vi "Frame.Dialog.vi"(6 "Signals":T1[](array[typedef]) {"Byte Order" items=["Little Endian", "Big Endian"]; "Data Type" items=["Signed", "Unsigned", "IEEE Float"]}, 7 "Show Name&ID":bool=TRUE, 8 "error in (no error)":errorcluster, 9 "ID":u16=1 caption="ID/Address" min=1 format="%.0x", 10 "Existing PIDs":string[](array[string]), 11 "Name":string) -> (0 "error out":errorcluster, 1 "ID out":u16=1 min=1 format="%.0x", 2 "Cancel PID?":bool, 3 "Name out":string, 4 "Signals out":T1[](array[typedef]) {"Byte Order" items=["Little Endian", "Big Endian"]; "Data Type" items=["Signed", "Unsigned", "IEEE Float"]})   [LabVIEW 2024, in "Diagnostics Addon System Explorer.lvlib"]
uses:
  Diagnostics Addon System Explorer.lvlib
  Addon Shared/Types/Signal.ctl
  <vilib>/NI/AMC/Create Single Message.vi
  <vilib>/NI/AMC/Update Message Routing Info.vi
  <vilib>/NI/AMC/Read Termination Message.vi
  Addon Shared/SubVIs/Constants.vi
  <vilib>/NI/AMC/Globals.vi
  <vilib>/NI/AMC/Send Message.vi
  Addon Shared/Diagnostics Addon Shared.lvlib
  <vilib>/NI/AMC/AMC.lvlib
panel:
  in  "Add":bool
  in  "Header":cluster{"Section Name":string}={"Section Name"="Frame Settings"}
  in  "SHDocVw.IWebBrowser":refnum<k7>(container)
  in  "Default":dbl format="%g"
  in  "Units":string
  in  "Endian":u8(ring) items=["Little", "Big"]
  in  "Datatype":u8(ring)=1 items=["Signed", "Unsigned", "Float"]
  in  "Remove":bool
  in  "Cancel":bool
  in  "OK":bool
  in  "Maximum":dbl=255.0 format="%g"
  in  "Minimum":dbl format="%g"
  in  "Offset":dbl format="%g"
  in  "Factor":dbl=1.0 format="%g"
  in  "Length":u32=8
  in  "Start Bit":u32
  in  "Signal Name":string
  in  "Signals":i32(listbox)
  in  "Cancel PID":bool
  in  "Apply":bool
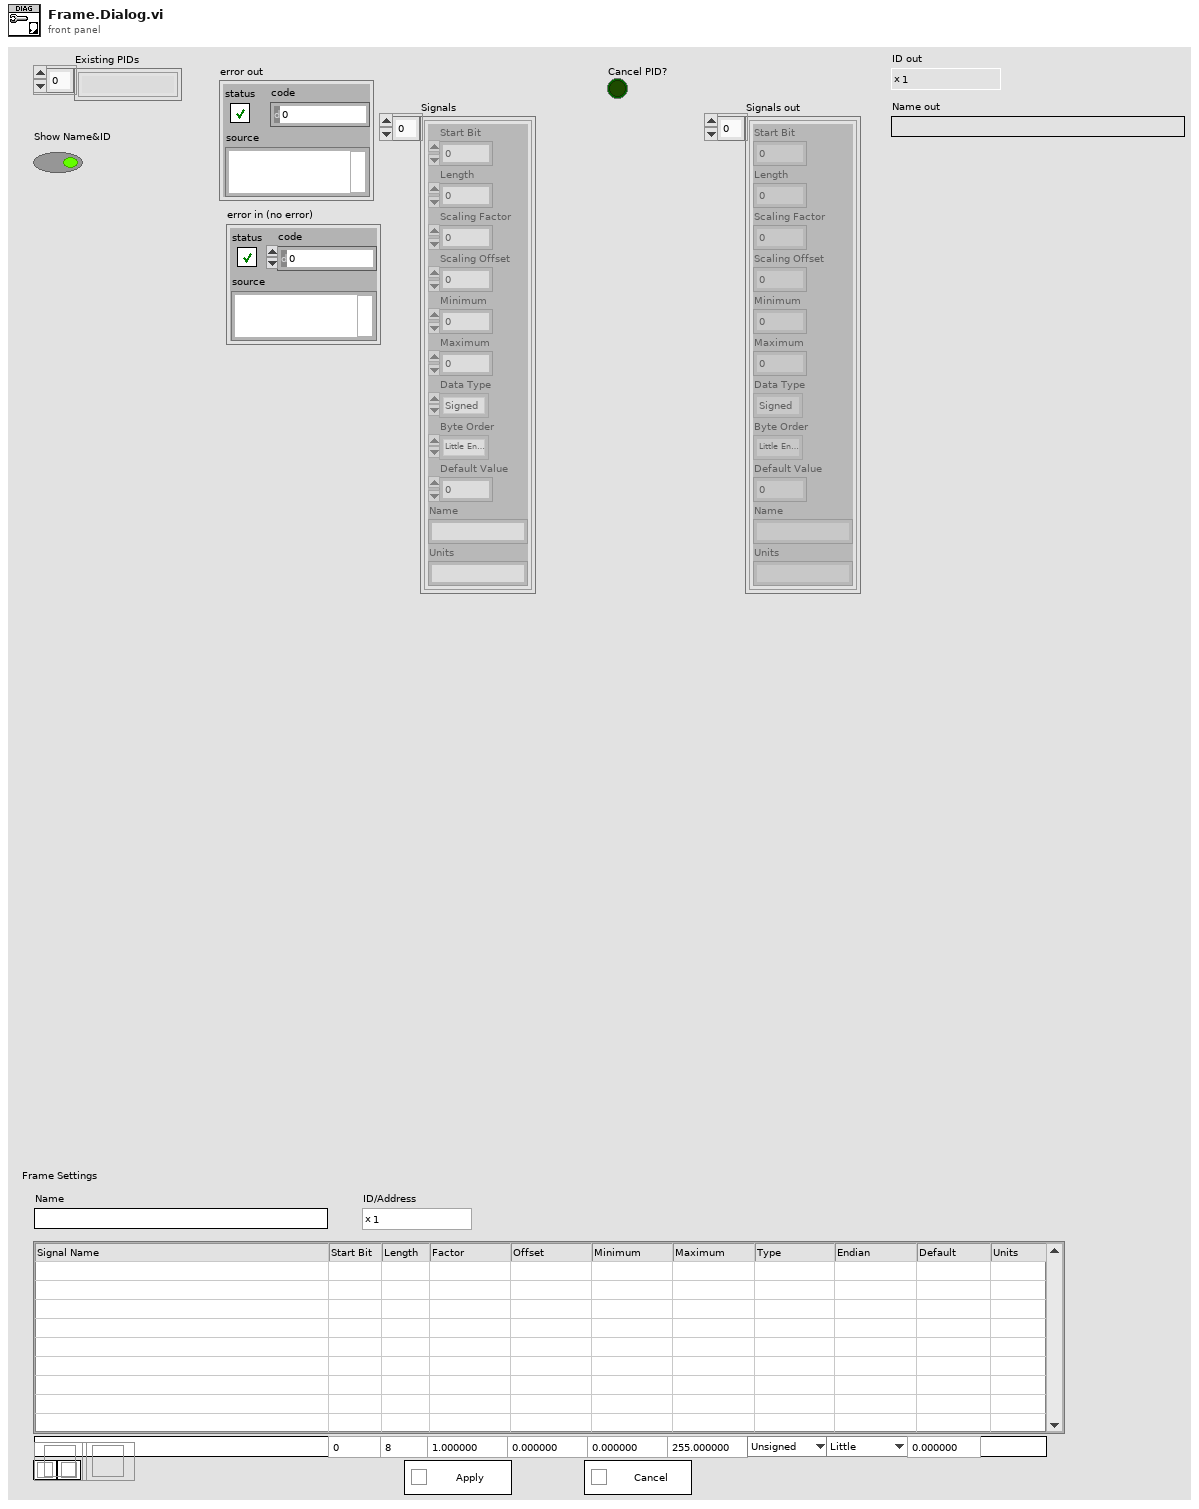
[diagram p1: front panel]
types:
  T1 = typedef "Diagnostics Addon Shared.lvlib/Signal.ctl" = cluster{"Start Bit":u32, "Length":u32, "Scaling Factor":dbl, "Scaling Offset":dbl, "Minimum":dbl, "Maximum":dbl, "Data Type":u32, "Byte Order":u32, "Default Value":dbl, "Name":string, "Units":string}
  T2 = cluster{"NewControlRefs":refnum<vi>[], "Add":refnum<vi>, "Listbox":refnum<vi>, "Remove":refnum<vi>, "Apply":refnum<vi>, "Cancel PID":refnum<vi>}
  T3 = typedef "AMC.lvlib/Message Queue.ctl" = refnum<queue>
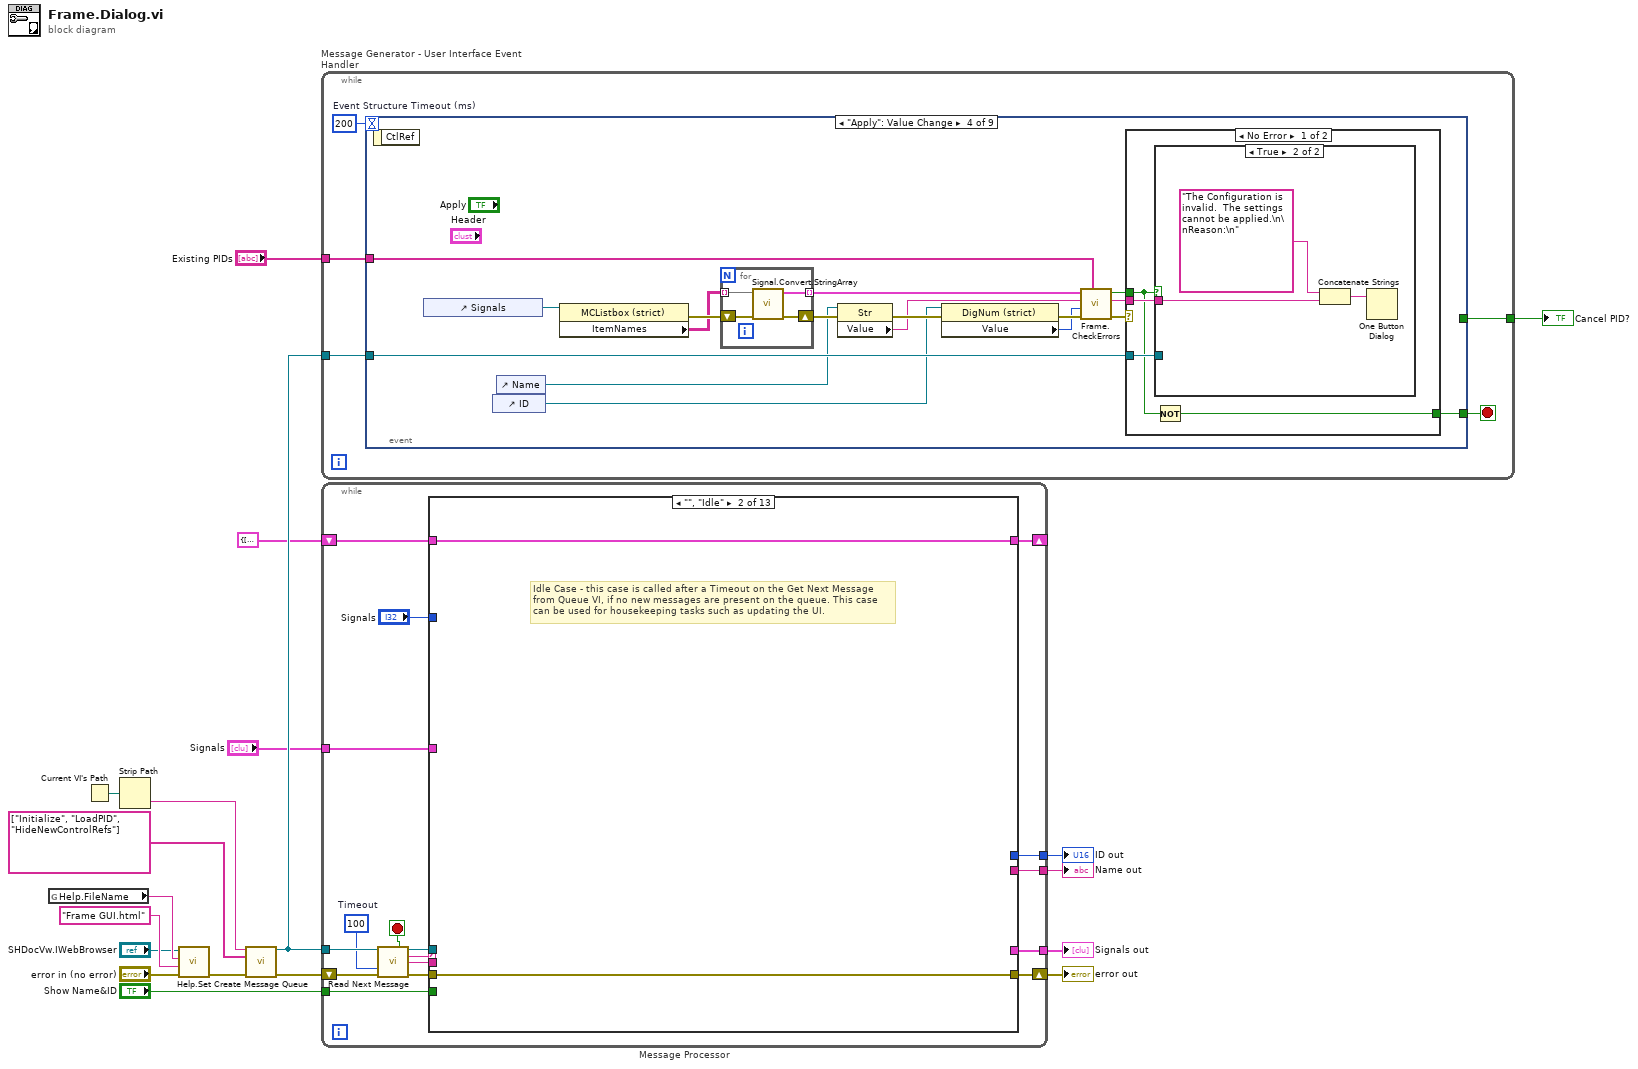
[diagram p0: block diagram]
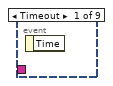
[diagram p2: hidden frame]
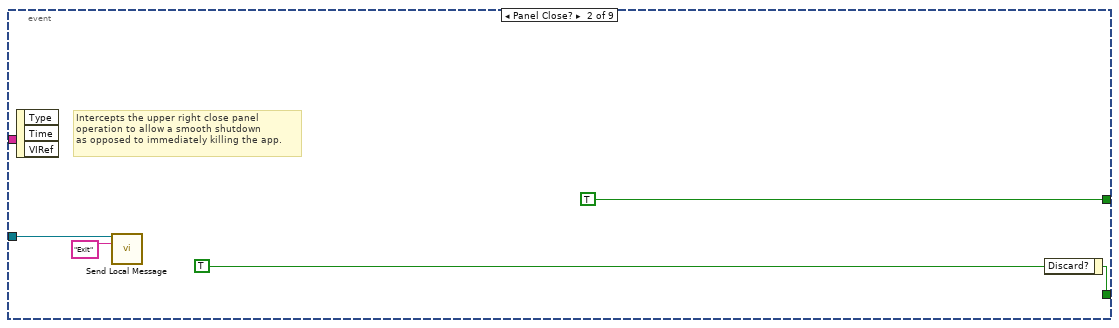
[diagram p3: hidden frame]
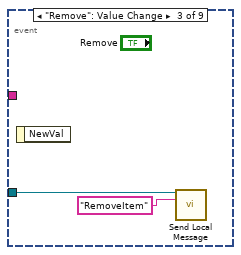
[diagram p4: hidden frame]
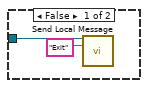
[diagram p5: hidden frame]
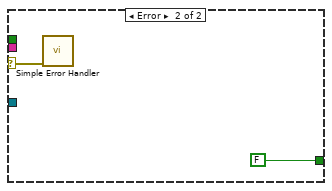
[diagram p6: hidden frame]
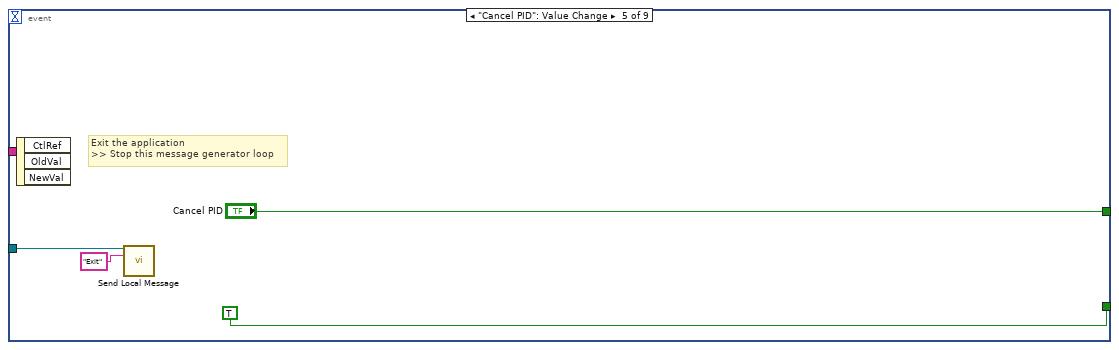
[diagram p7: hidden frame]
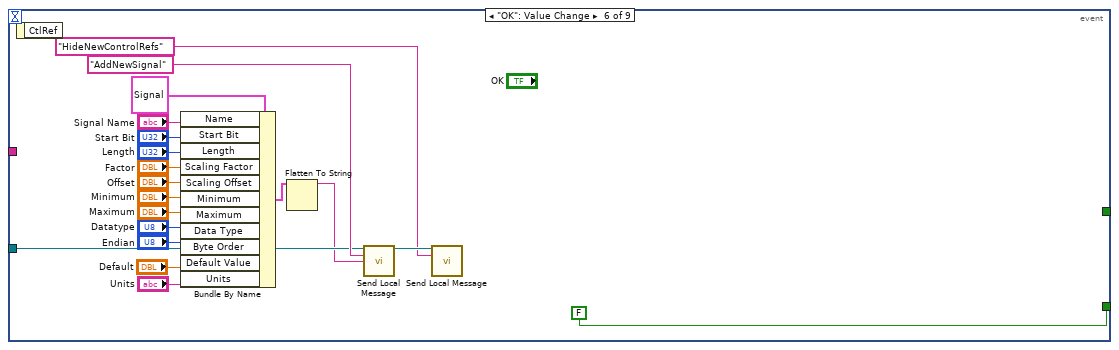
[diagram p8: hidden frame]
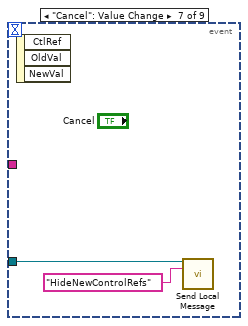
[diagram p9: hidden frame]
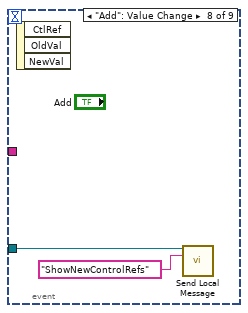
[diagram p10: hidden frame]
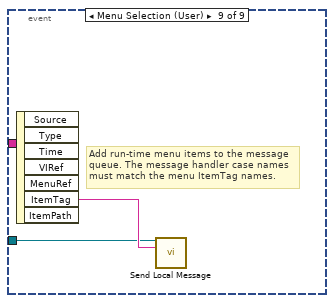
[diagram p11: hidden frame]
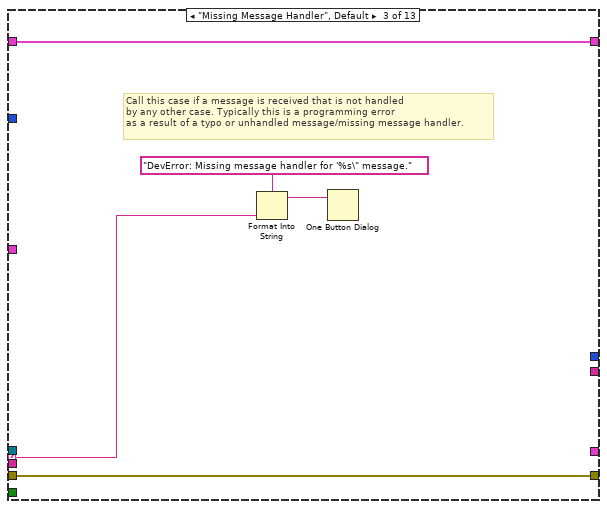
[diagram p13: hidden frame]
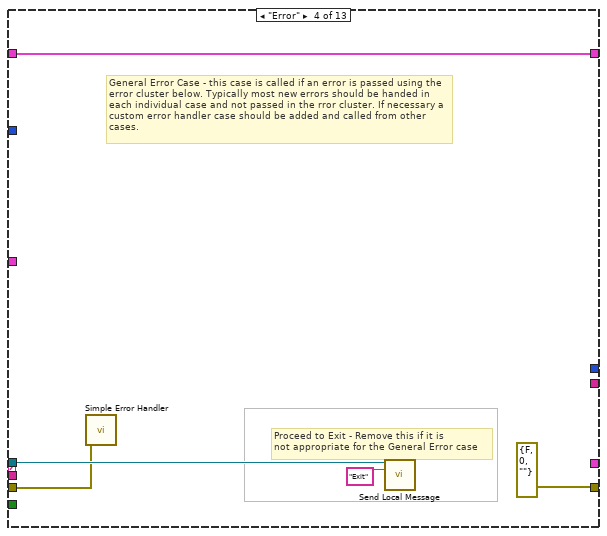
[diagram p14: hidden frame]
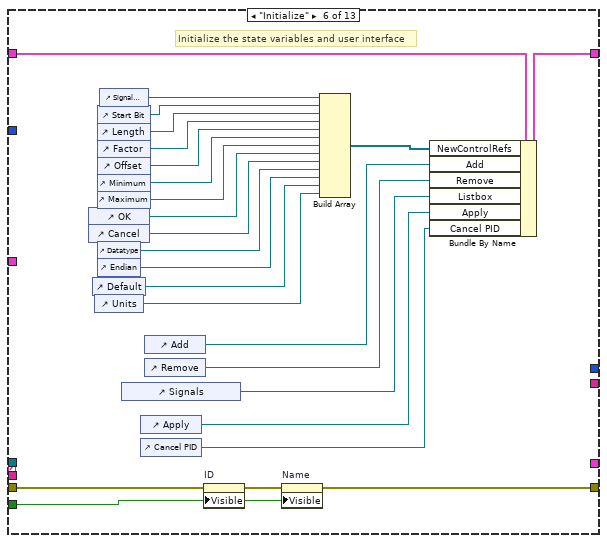
[diagram p16: hidden frame]
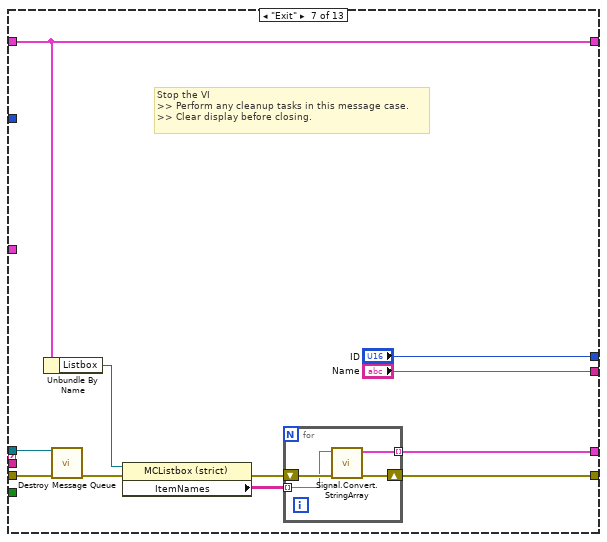
[diagram p17: hidden frame]
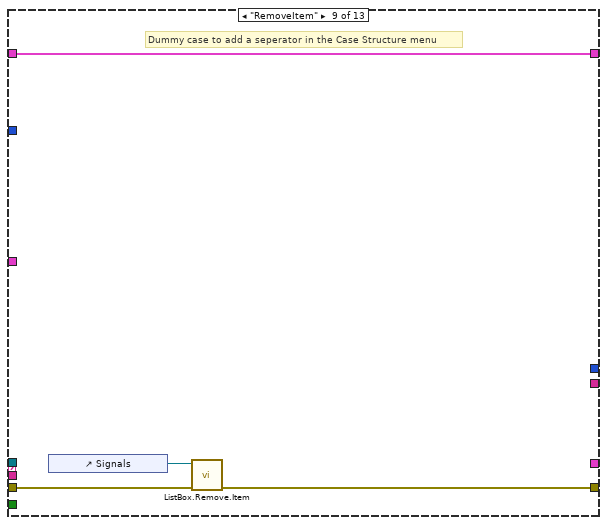
[diagram p19: hidden frame]
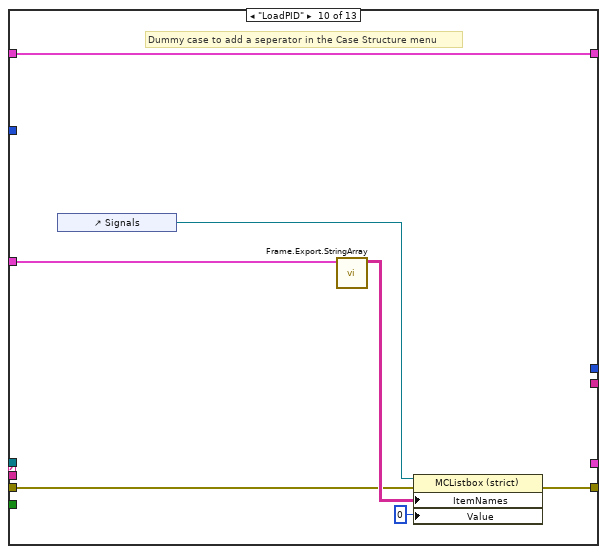
[diagram p20: hidden frame]
diagram:
  n1 = global read "Constants.vi" "Help.FileName"() -> (w4:string)
  n2 = Current VI's Path() -> (path=w15:path)
  n3 = Strip Path(path=w15) -> (name=w18:string)  [unwired: 1 out]
  n4 = call "Help.Set.vi"("error in (no error)"="error in (no error)", "HTML File"="Frame GUI.html", "Main CHM File"=w4, "SHDocVw.IWebBrowser2"="SHDocVw.IWebBrowser") -> ("error out"=w1:errorcluster)  [unwired: 7 in]
  n5 = call <vilib>:"Create Message Queue.vi"("message queue name"=w18, "initial message names"=string[] ["Initialize", "LoadPID", "HideNewControlRefs"], "error in"=w1) -> ("message queue out"=w17:T3, "error out"=w16:errorcluster)  [unwired: 11 in]
  n6 = while "Message Generator - User Interface Event Handler" {
    tunnel: w17 -> [w22]
    tunnel: [w21] -> w13
    tunnel: "Existing PIDs" -> [w20]
    stop <- w23 stop-if-true
    w24 = 200  # Event Structure Timeout (ms)
    n7 = event shown="[3] \"Apply\": Value Change" {
      selector: _ -> [_ _ _ _ _ _ _ _ _]
      dyn-events: _ -> [_ _ _ _ _ _ _ _ _]
      timeout: w24 -> [_ _ _ _ _ _ _ _ _]
      tunnel: [_ w28 _ w42 TRUE ("Discard?") FALSE ("Discard?") _ _ _] -> w23
      tunnel: w22 -> [_ w26 w29 w46 w64 w83 w86 w88 w90]
      tunnel: [_ TRUE ("Cancel PID") _ _ "Cancel PID" _ _ _ _] -> w21
      tunnel: w20 -> [_ _ _ w45 _ _ _ _ _]
      event Timeout {
        n8 = event-data() -> ()  [unwired: 2 out]
      }
      event Panel Close? {
        w28 = TRUE ("Discard?")
        # "Intercepts the upper right close panel\noperation to allow a smooth shutdown\nas opposed to immediately killing the app."
        n9 = event-data() -> ()  [unwired: 4 out]
        n10 = call <vilib>:"Send Local Message.vi"("message queue in"=w26, "message name"="Exit") -> ()  [unwired: 11 in, 3 out]
        n11 = event-data("Discard?"=w28) -> ()  [unwired: 1 in, 1 out]
      }
      event "Remove": Value Change {
        n12 = event-data() -> ()  [unwired: 2 out]
        n13 = call <vilib>:"Send Local Message.vi"("message queue in"=w29, "message name"="RemoveItem") -> ()  [unwired: 11 in, 3 out]
      }
      event "Apply": Value Change {
        n14 = event-data() -> ()  [unwired: 2 out]
        n15 = control-ref of="Signals"() -> (w40:refnum<vi>)
        n16 = control-ref of="ID"() -> (w33:refnum<vi>)
        n17 = control-ref of="Name"() -> (w34:refnum<vi>)
        n18 = property class="MCListbox (strict)"(reference=w40) -> (error out=w41:errorcluster, "ItemNames"=w39:string[][])  [unwired: 1 in, 1 out]
        n19 = for {
          shift-right: [w50] -> w37
          shift-left: w41 -> [w51]
          tunnel: w39 -> [w49] mode=indexing
          tunnel: [w48] -> w38 mode=indexing
          n20 = call "Signal.Convert.StringArray.vi"("error in (no error)"=w51, "Signal Parameters"=w49) -> ("error out"=w50:errorcluster, "Signal Parameters"=w48:T1)  [unwired: 8 in]
        }
        n21 = property class="Str"(reference=w34, error in=w37) -> (error out=w36:errorcluster, "Value"=w31:string)  [unwired: 1 out]
        n22 = property class="DigNum (strict)"(reference=w33, error in=w36) -> (error out=w35:errorcluster, "Value"=w32:u16)  [unwired: 1 out]
        n23 = call "Frame.CheckErrors.vi"("Existing PIDs"=w45, "error in (no error)"=w35, "ID"=w32, "Name"=w31, "Signals"=w38) -> ("error out"=w43:errorcluster, "Error Type"=w44:string, "Error?"=w47:bool)  [unwired: 4 in]
        n24 = case shown="No Error" w43 {
          selector: w43 -> [_ w62]
          tunnel: w47 -> [w53 _]
          tunnel: w46 -> [w55 _]
          tunnel: w44 -> [w54 _]
          tunnel: [w52 FALSE] -> w42
          frame No Error {
            n25 = case shown="True" w53 {
              tunnel: w55 -> [w57 _]
              tunnel: w54 -> [_ w60]
              frame False {
                n26 = call <vilib>:"Send Local Message.vi"("message queue in"=w57, "message name"="Exit" ("Message Name")) -> ()  [unwired: 11 in, 3 out]
              }
              frame True {
                n27 = Concatenate Strings("The Configuration is invalid.  The settings cannot be applied.\n\nReason:\n" ("message"), w60) -> (w58:string)
                n28 = One Button Dialog(message=w58) -> ()  [unwired: 1 in, 1 out]
              }
            }
            n29 = Not(x=w53) -> (.not. x?=w52:bool)
          }
          frame Error {
            n30 = call <vilib>:"Simple Error Handler.vi"("error in (no error)"=w62) -> ()  [unwired: 4 in, 5 out]
          }
        }
      }
      event "Cancel PID": Value Change {
        # "Exit the application\n>> Stop this message generator loop"
        n31 = event-data() -> ()  [unwired: 4 out]
        n32 = call <vilib>:"Send Local Message.vi"("message queue in"=w64, "message name"="Exit") -> ()  [unwired: 11 in, 3 out]
      }
      event "OK": Value Change {
        n33 = event-data() -> ()  [unwired: 2 out]
        n34 = Bundle By Name(cluster=T1 {"Start Bit"=0, "Length"=0, "Scaling Factor"=0.0, "Scaling Offset"=0.0, "Minimum"=0.0, "Maximum"=0.0, "Data Type"=0, "Byte Order"=0, "Default Value"=0.0, "Name"="", "Units"=""} ("Signal Parameters"), "Name"="Signal Name", "Start Bit"="Start Bit", "Length"="Length", "Scaling Factor"="Factor", "Scaling Offset"="Offset", "Minimum"="Minimum", "Maximum"="Maximum", "Data Type"="Datatype", "Byte Order"="Endian", "Default Value"="Default", "Units"="Units") -> (w74:T1)
        n35 = Flatten To String(anything=w74) -> (data string=w73:string)  [unwired: 3 in, 2 out]
        n36 = call <vilib>:"Send Local Message.vi"("message queue in"=w83, "message name"="AddNewSignal", "message value"=w73) -> ("message queue out"=w72:T3)  [unwired: 10 in, 2 out]
        n37 = call <vilib>:"Send Local Message.vi"("message queue in"=w72, "message name"="HideNewControlRefs" ("Message Name")) -> ()  [unwired: 11 in, 3 out]
      }
      event "Cancel": Value Change {
        n38 = event-data() -> ()  [unwired: 4 out]
        n39 = call <vilib>:"Send Local Message.vi"("message queue in"=w86, "message name"="HideNewControlRefs" ("Message Name")) -> ()  [unwired: 11 in, 3 out]
      }
      event "Add": Value Change {
        n40 = event-data() -> ()  [unwired: 4 out]
        n41 = call <vilib>:"Send Local Message.vi"("message queue in"=w88, "message name"="ShowNewControlRefs" ("Message Name")) -> ()  [unwired: 11 in, 3 out]
      }
      event Menu Selection (User) {
        # "Add run-time menu items to the message\nqueue. The message handler case names must match the menu ItemTag names."
        n42 = event-data() -> ("ItemTag"=w91:string)  [unwired: 7 out]
        n43 = call <vilib>:"Send Local Message.vi"("message queue in"=w90, "message name"=w91) -> ()  [unwired: 11 in, 3 out]
      }
    }
  }
  "Cancel PID?" <- w13
  n44 = while "Message Processor" {
    shift-left: w16 -> [w102]
    shift-right: [w106] -> w12
    tunnel: w17 -> [w103]
    shift-left: T2 {"NewControlRefs"=[], "Add"=refnum, "Listbox"=refnum, "Remove"=refnum, "Apply"=refnum, "Cancel PID"=refnum} ("State Variables") -> [w108]
    shift-right: [w107] -> _
    tunnel: "Signals" -> [w96]
    tunnel: [w95] -> w9
    tunnel: [w94] -> w8
    tunnel: [w93] -> w7
    tunnel: "Show Name&ID" -> [w92]
    stop <- w105 stop-if-true
    w100 = 100  # Timeout
    n45 = call <vilib>:"Read Next Message.vi"("message queue in"=w103, "timeout (1 ms)"=w100, "error in"=w102) -> ("exit process?"=w105:bool, "message queue out"=w104:T3, "message name"=w99:string, "message value"=w98:string, "error out"=w101:errorcluster)  [unwired: 5 in, 3 out]
    n46 = case shown="\"\", \"Idle\"" w99 {
      selector: w99 -> [_ _ w115 _ _ _ _ _ _ _ _ _ _]
      tunnel: [w110 w112 w117 w122 w124 w138 w158 w166 w170 w177 w183 w200 w214] -> w107
      tunnel: w108 -> [w110 w112 w117 w122 w124 w139 w158 w166 w170 w177 w183 w200 w214]
      tunnel: w104 -> [_ _ _ w120 _ _ w159 _ _ _ _ _ _]
      tunnel: w101 -> [w109 w111 w116 w118 w123 w129 w160 w165 w168 w171 w186 w199 w213]
      tunnel: [w109 w111 w116 errorcluster {"status"=FALSE, "code"=0, "source"=""} ("error out") w123 w128 w153 w165 w167 w174 w180 w189 w204] -> w106
      tunnel: w98 -> [_ _ _ _ _ _ _ _ _ _ w185 _ _]
      tunnel: "Signals" -> [_ _ _ _ _ _ _ _ _ _ _ _ _]
      tunnel: w96 -> [_ _ _ _ _ _ _ _ _ w172 _ _ _]
      tunnel: [_ _ _ _ _ _ w152 _ _ _ _ _ _] -> w95
      tunnel: [_ _ _ _ _ _ "Name" _ _ _ _ _ _] -> w94
      tunnel: [_ _ _ _ _ _ "ID" _ _ _ _ _ _] -> w93
      tunnel: w92 -> [_ _ _ _ _ w127 _ _ _ _ _ _ _]
      frame "---------- Framework Operations ----------" {
        # "Dummy case to add a seperator in the Case Structure menu"
      }
      frame "", "Idle" {
        # "Idle Case - this case is called after a Timeout on the Get Next Message from Queue VI, if no new messages are present on the queue. This case can be used for housekeeping tasks such as updating the UI."
      }
      frame "Missing Message Handler", Default {
        # "Call this case if a message is received that is not handled \nby any other case. Typically this is a programming error\nas a result of a typo or unhandled message/missing message handler."
        n47 = Format Into String(format string="DevError: Missing message handler for '%s\" message." ("message"), w115) -> (resulting string=w113:string)  [unwired: 2 in, 1 out]
        n48 = One Button Dialog(message=w113) -> ()  [unwired: 2 out]
      }
      frame "Error" {
        # "Proceed to Exit - Remove this if it is\nnot appropriate for the General Error case"
        # "General Error Case - this case is called if an error is passed using the error cluster below. Typically most new errors should be handed in each individual case and not passed in the rror cluster. If necessary a custom error handler case should be added and called from other cases."
        n49 = call <vilib>:"Simple Error Handler.vi"("error in (no error)"=w118) -> ()  [unwired: 1 in, 8 out]
        n50 = call <vilib>:"Send Local Message.vi"("message queue in"=w120, "message name"="Exit") -> ()  [unwired: 11 in, 3 out]
      }
      frame "---------- Generic Operations ----------" {
        # "Dummy case to add a seperator in the Case Structure menu"
      }
      frame "Initialize" {
        # "Initialize the state variables and user interface"
        n51 = control-ref of="OK"() -> (w148:refnum<vi>)
        n52 = control-ref of="Cancel"() -> (w149:refnum<vi>)
        n53 = control-ref of="Default"() -> (w126:refnum<vi>)
        n54 = control-ref of="Units"() -> (w125:refnum<vi>)
        n55 = control-ref of="Start Bit"() -> (w142:refnum<vi>)
        n56 = control-ref of="Length"() -> (w143:refnum<vi>)
        n57 = control-ref of="Factor"() -> (w144:refnum<vi>)
        n58 = control-ref of="Offset"() -> (w145:refnum<vi>)
        n59 = control-ref of="Minimum"() -> (w146:refnum<vi>)
        n60 = control-ref of="Maximum"() -> (w147:refnum<vi>)
        n61 = control-ref of="Datatype"() -> (w134:refnum<vi>)
        n62 = control-ref of="Endian"() -> (w133:refnum<vi>)
        n63 = control-ref of="Signal Name"() -> (w141:refnum<vi>)
        n64 = control-ref of="Signals"() -> (w136:refnum<vi>)
        n65 = control-ref of="Apply"() -> (w132:refnum<vi>)
        n66 = control-ref of="Cancel PID"() -> (w131:refnum<vi>)
        n67 = control-ref of="Add"() -> (w137:refnum<vi>)
        n68 = control-ref of="Remove"() -> (w135:refnum<vi>)
        n69 = property on="ID" class="DigNum (strict)"(error in=w129, "Visible"=w127) -> (error out=w130:errorcluster)  [unwired: 1 in, 1 out]
        n70 = property on="Name" class="Str"(error in=w130, "Visible"=w127) -> (error out=w128:errorcluster)  [unwired: 1 in, 1 out]
        n71 = Build Array(w141, w142, w143, w144, w145, w146, w147, w148, w149, w134, w133, w126, w125) -> (w140:refnum<vi>[])
        n72 = Bundle By Name(cluster=w139, "NewControlRefs"=w140, "Add"=w137, "Remove"=w135, "Listbox"=w136, "Apply"=w132, "Cancel PID"=w131) -> (w138:T2)
      }
      frame "Exit" {
        # "Stop the VI\n>> Perform any cleanup tasks in this message case.\n>> Clear display before closing."
        n73 = Unbundle By Name(w158) -> ("Listbox"=w157:refnum<vi>)
        n74 = call <vilib>:"Destroy Message Queue.vi"("message queue in"=w159, "error in"=w160) -> ("error out"=w156:errorcluster)  [unwired: 11 in, 2 out]
        n75 = property class="MCListbox (strict)"(reference=w157, error in=w156) -> (error out=w154:errorcluster, "ItemNames"=w155:string[][])  [unwired: 1 out]
        n76 = for {
          shift-right: [w163] -> w153
          shift-left: w154 -> [w164]
          tunnel: w155 -> [w162] mode=indexing
          tunnel: [w161] -> w152 mode=indexing
          n77 = call "Signal.Convert.StringArray.vi"("error in (no error)"=w164, "Signal Parameters"=w162) -> ("error out"=w163:errorcluster, "Signal Parameters"=w161:T1)  [unwired: 8 in]
        }
      }
      frame "---------- Application Operations ----------" {
        # "Dummy case to add a seperator in the Case Structure menu"
      }
      frame "RemoveItem" {
        # "Dummy case to add a seperator in the Case Structure menu"
        n78 = control-ref of="Signals"() -> (w169:refnum<vi>)
        n79 = call "ListBox.Remove.Item.vi"("error in (no error)"=w168, "MulticolumnListbox in"=w169) -> ("error out"=w167:errorcluster)  [unwired: 9 in]
      }
      frame "LoadPID" {
        # "Dummy case to add a seperator in the Case Structure menu"
        n80 = control-ref of="Signals"() -> (w176:refnum<vi>)
        n81 = call "Frame.Export.StringArray.vi"("Frame Parameters"=w172) -> ("Frame Parameters"=w173:string[][])  [unwired: 9 in, 1 out]
        n82 = property class="MCListbox (strict)"(reference=w176, error in=w171, "ItemNames"=w173, "Value"=0) -> (error out=w174:errorcluster)  [unwired: 1 out]
      }
      frame "AddNewSignal" {
        # "Dummy case to add a seperator in the Case Structure menu"
        n83 = Unflatten From String(type=T1 {"Start Bit"=0, "Length"=0, "Scaling Factor"=0.0, "Scaling Offset"=0.0, "Minimum"=0.0, "Maximum"=0.0, "Data Type"=0, "Byte Order"=0, "Default Value"=0.0, "Name"="", "Units"=""} ("Signal Parameters"), binary string=w185, error in (no error)=w186) -> (value=w179:T1, error out=w181:errorcluster)  [unwired: 2 in, 1 out]
        n84 = Unbundle By Name(w183) -> ("Listbox"=w182:refnum<vi>)
        n85 = call "Signal.Export.StringArray.vi"("Signal Parameters"=w179) -> ("Array"=w178:string[])  [unwired: 10 in]
        n86 = call "Listbox.Add.Item.vi"("error in (no error)"=w181, "Item"=w178, "MulticolumnListbox in"=w182) -> ("error out"=w180:errorcluster)  [unwired: 8 in]
      }
      frame "HideNewControlRefs" {
        w191 = TRUE ("Visible")
        # "Dummy case to add a seperator in the Case Structure menu"
        n87 = Unbundle By Name(w200) -> ("Cancel PID"=w187:refnum<vi>, "Apply"=w188:refnum<vi>, "Remove"=w193:refnum<vi>, "Add"=w195:refnum<vi>, "NewControlRefs"=w198:refnum<vi>[])
        n88 = call "Controls.Set.Visible.vi"("error in"=w199, "Visible?"=FALSE, "Control Refs"=w198) -> ("error out"=w196:errorcluster)  [unwired: 8 in]
        n89 = property class="Bool"(reference=w195, error in=w196, "Visible"=w191) -> (error out=w194:errorcluster)  [unwired: 1 out]
        n90 = property class="Bool"(reference=w193, error in=w194, "Visible"=w191) -> (error out=w190:errorcluster)  [unwired: 1 out]
        n91 = property class="Bool"(reference=w188, error in=w190, "Visible"=w191) -> (error out=w192:errorcluster)  [unwired: 1 out]
        n92 = property class="Bool"(reference=w187, error in=w192, "Visible"=w191) -> (error out=w189:errorcluster)  [unwired: 1 out]
      }
      frame "ShowNewControlRefs" {
        w203 = FALSE ("Visible")
        # "Dummy case to add a seperator in the Case Structure menu"
        n93 = Unbundle By Name(w214) -> ("Apply"=w202:refnum<vi>, "Cancel PID"=w201:refnum<vi>, "Remove"=w207:refnum<vi>, "Add"=w209:refnum<vi>, "NewControlRefs"=w212:refnum<vi>[])
        n94 = call "Controls.Set.Visible.vi"("error in"=w213, "Visible?"=TRUE, "Control Refs"=w212) -> ("error out"=w210:errorcluster)  [unwired: 8 in]
        n95 = property class="Bool"(reference=w209, error in=w210, "Visible"=w203) -> (error out=w208:errorcluster)  [unwired: 1 out]
        n96 = property class="Bool"(reference=w207, error in=w208, "Visible"=w203) -> (error out=w205:errorcluster)  [unwired: 1 out]
        n97 = property class="Bool"(reference=w201, error in=w205, "Visible"=w203) -> (error out=w206:errorcluster)  [unwired: 1 out]
        n98 = property class="Bool"(reference=w202, error in=w206, "Visible"=w203) -> (error out=w204:errorcluster)  [unwired: 1 out]
      }
    }
  }
  "error out" <- w12
  "Signals out" <- w9
  "ID out" <- w7
  "Name out" <- w8
